vi "Pose_getXYAngle.vi"(11 "in POSE":T1 {"ROTATION"."SIN" format="%13.4f"; "ROTATION"."COS" format="%13.4f"; "ROTATION"."VALUE" format="%13.4f"; "TRANSLATION"."Y" format="%14.3f"; "TRANSLATION"."X" format="%14.3f"}) -> (1 "Angle":dbl, 2 "Y":dbl, 3 "X":dbl)   [LabVIEW 2019, in "Trajectory_Library.lvlib"]
doc: "Returns the X, Y, Angle components of the pose.\n\nParmeters:\n- IN POSE - The POSE data structure\n\nRETURNS:\n - X - X translation value\n - Y - Y translation value\n - Rotataion angle value"
uses:
  POSE2D.ctl
  TRANSLATION2D.ctl
  ROTATION2D.ctl
  Trajectory_Library.lvlib
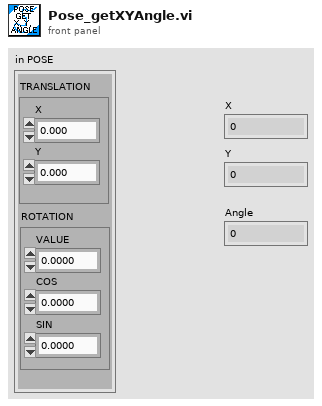
[diagram p1: front panel]
types:
  T1 = typedef "Trajectory_Library.lvlib/POSE2D.ctl" = cluster{"TRANSLATION":T2, "ROTATION":T3}
  T2 = typedef "Trajectory_Library.lvlib/TRANSLATION2D.ctl" = cluster{"X":dbl, "Y":dbl}
  T3 = typedef "Trajectory_Library.lvlib/ROTATION2D.ctl" = cluster{"VALUE":dbl, "COS":dbl, "SIN":dbl}
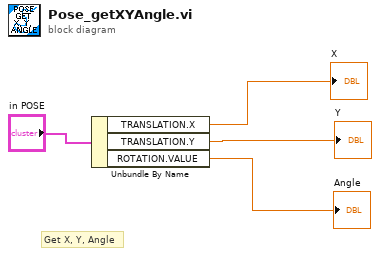
[diagram p0: block diagram]
diagram:
  # "Get X, Y, Angle"
  n1 = Unbundle By Name("in POSE") -> ("TRANSLATION.X"=→"X":dbl, "TRANSLATION.Y"=→"Y":dbl, "ROTATION.VALUE"=→"Angle":dbl)
